vi "p1.vi"() -> ()   [LabVIEW 2023, in "d5.lvlib"]
uses:
  d5.lvlib
  <vilib>/regexp/Match Regular Expression.xnode
  AOC/AOC.lvlib
panel:
  out "Answer":i64
  in  "Example":string="seeds: 79 14 55 13\n\nseed-to-soil map:\n50 98 2\n52 50 48\n\nsoil-to-fertilizer map:\n0 15 37\n37 52 2\n39 0 15\n\nfertilizer-to-water map:\n49 53 8\n0 11 42\n42 0 7\n57 7 4\n\nwater-to-light map:\n88 18 7\n18 25 70\n\nlight-to-temperature map:\n45 77 23\n81 45 19\n68 64 13\n\ntemperature-to-humidity map:\n0 69 1\n1 0 69\n\nhumidity-to-location map:\n60 56 37\n56 93 4"
  in  "Example":bool
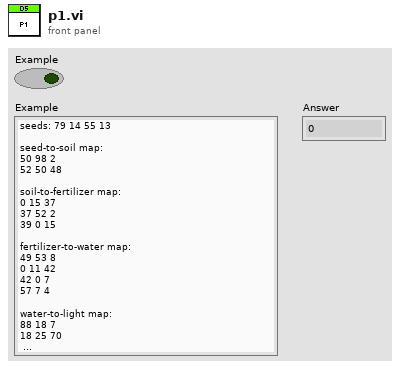
[diagram p1: front panel]
types:
  T1 = cluster{cluster{"dst":i64, "src":i64, "rng":i64}[]}
  T2 = cluster{cluster{"dst":i64, "src":i64, "rng":i64}[]}[]
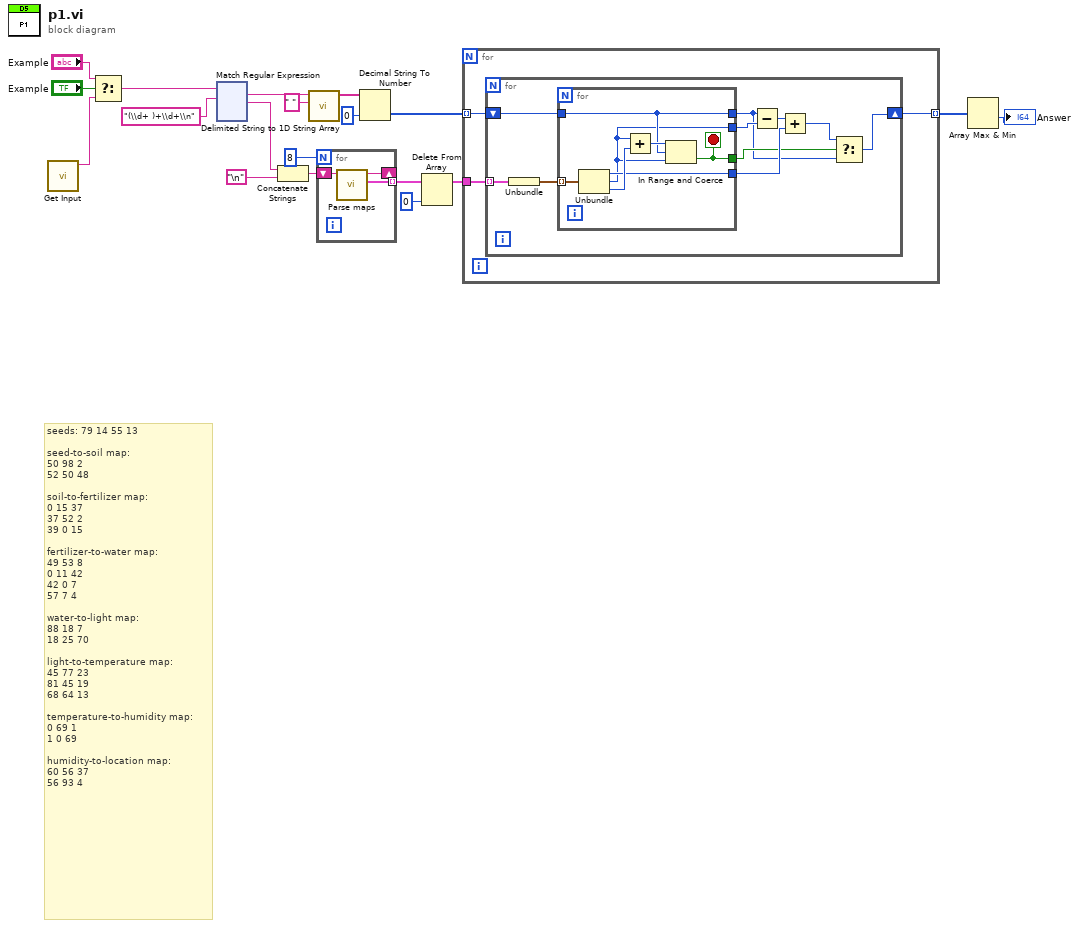
[diagram p0: block diagram]
diagram:
  # "seeds: 79 14 55 13\n\nseed-to-soil map:\n50 98 2\n52 50 48\n\nsoil-to-fertilizer map:\n0 15 37\n37 52 2\n39 0 15\n\nfertilizer-to-water map:\n49 53 8\n0 11 42\n42 0 7\n57 7 4\n\nwater-to-light map:\n88 18 7\n18 25 70\n\nlight-to-temperature map:\n45 77 23\n81 45 19\n68 64 13\n\ntemperature-to-humidity map:\n0 69 1\n1 0 69\n\nhumidity-to-location map:\n60 56 37\n56 93 4"
  n1 = call "Get Input.vi"() -> ("Input"=w1:string)  [unwired: 11 in]
  n2 = Select(t="Example", s="Example", f=w1) -> (s? t:f=w12:string)
  n3 = xnode "Match Regular Expression"("input string"=w12, "regular expression"="(\\d+ )+\\d+\\n") -> ("whole match"=w11:string, "after match"=w10:string)  [unwired: 4 in, 3 out]
  n4 = Concatenate Strings(w10, "\n") -> (w14:string)
  n5 = call <vilib>:"Delimited String to 1D String Array.vi"("delimiter"=" ", "delimited string"=w11) -> ("string array"=w9:string[])  [unwired: 9 in]
  n6 = for {
    N: 8 -> [_]
    shift-right: [w21] -> _
    shift-left: w14 -> [w22]
    tunnel: [w20] -> w7 mode=indexing
    n7 = call "Parse maps.vi"("string in"=w22) -> ("map"=w20:T1, "string out"=w21:string)  [unwired: 9 in]
  }
  n8 = Decimal String To Number(string=w9, default (0L)=i64 0 ("default (0 I32)")) -> (number=w8:i64[])  [unwired: 1 in, 1 out]
  n9 = Delete From Array(array=w7, index=0) -> (array with subset deleted=w6:T2)  [unwired: 1 in, 1 out]
  n10 = for {
    tunnel: w8 -> [w24] mode=indexing
    tunnel: w6 -> [w25]
    tunnel: [w23] -> w4 mode=indexing
    n11 = for {
      tunnel: w25 -> [w35] mode=indexing
      shift-right: [w26] -> w23
      shift-left: w24 -> [w34]
      n12 = Unbundle(w35) -> (w33:cluster{"dst":i64, "src":i64, "rng":i64}[])
      n13 = for {
        tunnel: w34 -> [w39]
        tunnel: w33 -> [w42] mode=indexing
        tunnel: [w39] -> w28
        tunnel: [w38] -> w31
        tunnel: [w37] -> w30
        tunnel: [w36] -> w29
        stop <- w36 stop-if-true
        n14 = Unbundle(w42) -> ("dst"=w38:i64, "src"=w37:i64, "rng"=w41:i64)
        n15 = Add(x=w37, y=w41) -> (x+y=w40:i64)
        n16 = In Range and Coerce(upper limit=w40, x=w39, lower limit=w37) -> (In Range?=w36:bool)  [unwired: 1 out]
      }
      n17 = Subtract(x=w28, y=w30) -> (x-y=w32:i64)
      n18 = Add(x=w32, y=w31) -> (x+y=w27:i64)
      n19 = Select(t=w27, s=w29, f=w28) -> (s? t:f=w26:i64)
    }
  }
  n20 = Array Max & Min(array=w4) -> (min value=→"Answer":i64)  [unwired: 3 out]
